vi "importExcel.vi"(1 "RANGE":string="A1:D2", 2 "Path":path) -> (0 "Excel Data":dbl[][](array[numeric]))   [LabVIEW 2019]
panel:
  in  "Array - Used for data type":string[][](array[string])
  in  "Excel._Worksheet 2":refnum<k7>
  in  "Excel._Application":refnum<k7>
  # "Filepath to Excel file"
  # "Specify range to import from Excel"
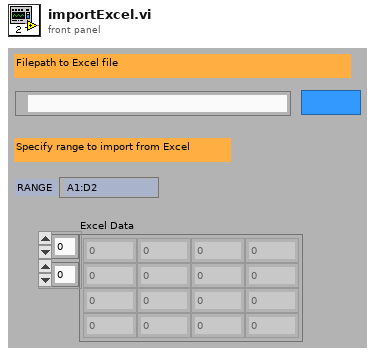
[diagram p1: front panel]
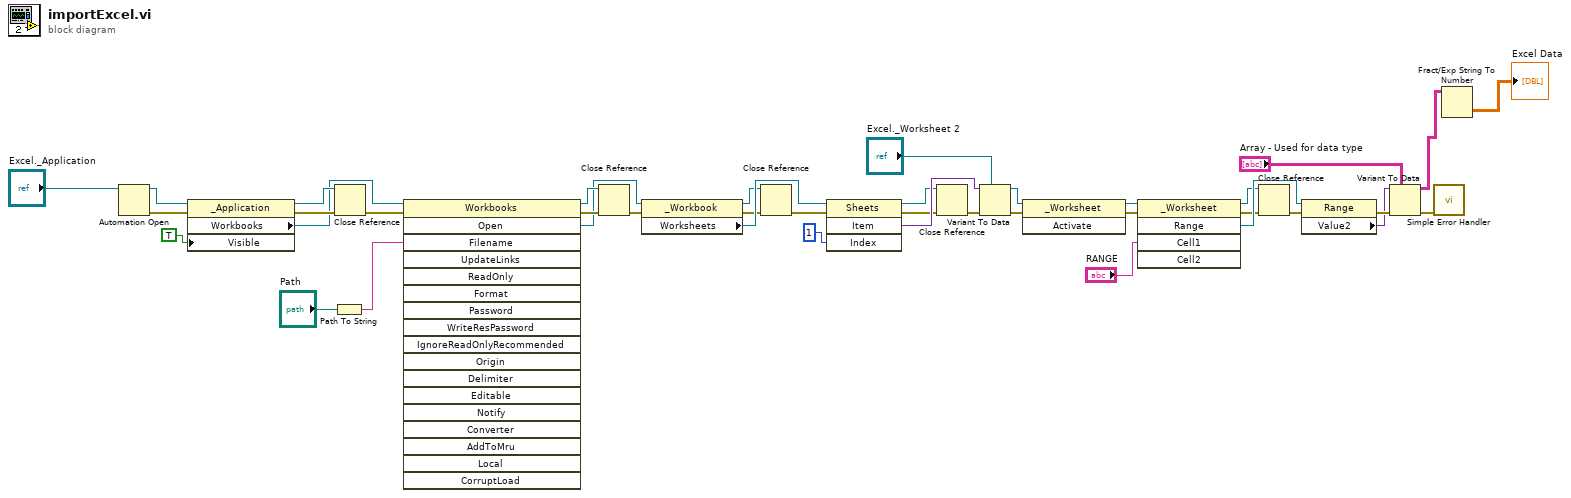
[diagram p0: block diagram]
diagram:
  n1 = Automation Open(Automation Refnum="Excel._Application") -> (Automation Refnum=w4:refnum<k7>, error out=w26:errorcluster)  [unwired: 3 in]
  n2 = property class="_Application"(reference=w4, error in=w26, "Visible"=TRUE) -> (reference out=w24:refnum<k7>, error out=w20:errorcluster, "Workbooks"=w11:refnum<k7>)
  n3 = Path To String(path="Path") -> (string=w38:string)
  n4 = Close Reference(reference=w24, error in (no error)=w20) -> (error out=w19:errorcluster)
  n5 = invoke class="Workbooks" method="Open"(reference=w11, error in=w19, "Filename"=w38) -> (reference out=w23:refnum<k7>, error out=w18:errorcluster, "Open"=w10:refnum<k7>)  [unwired: 15 in, 15 out]
  n6 = Close Reference(reference=w23, error in (no error)=w18) -> (error out=w17:errorcluster)
  n7 = property class="_Workbook"(reference=w10, error in=w17) -> (reference out=w22:refnum<k7>, error out=w16:errorcluster, "Worksheets"=w34:refnum<k7>)
  n8 = Close Reference(reference=w22, error in (no error)=w16) -> (error out=w15:errorcluster)
  n9 = invoke class="Sheets" method="Item"(reference=w34, error in=w15, "Index"=1) -> (reference out=w21:refnum<k7>, error out=w14:errorcluster, "Item"=w35:variant)  [unwired: 1 in, 1 out]
  n10 = Close Reference(reference=w21, error in (no error)=w14) -> (error out=w13:errorcluster)
  n11 = Variant To Data(error in=w13, type="Excel._Worksheet 2", Variant=w35) -> (data=w5:refnum<k7>, error out=w25:errorcluster)
  n12 = invoke class="_Worksheet" method="Activate"(reference=w5, error in=w25) -> (reference out=w3:refnum<k7>, error out=w12:errorcluster)  [unwired: 1 in, 1 out]
  n13 = invoke class="_Worksheet" method="Range"(reference=w3, error in=w12, "Cell1"="RANGE") -> (reference out=w9:refnum<k7>, error out=w8:errorcluster, "Range"=w29:refnum<k7>)  [unwired: 2 in, 2 out]
  n14 = Close Reference(reference=w9, error in (no error)=w8) -> (error out=w7:errorcluster)
  n15 = property class="Range"(reference=w29, error in=w7) -> (error out=w31:errorcluster, "Value2"=w30:variant)  [unwired: 1 out]
  n16 = Variant To Data(error in=w31, type="Array - Used for data type", Variant=w30) -> (data=w2:string[][], error out=w6:errorcluster)
  n17 = call <vilib>:"Simple Error Handler.vi"("error in (no error)"=w6) -> ()  [unwired: 4 in, 5 out]
  n18 = Fract/Exp String To Number(string=w2) -> (number=→"Excel Data":dbl[][])  [unwired: 3 in, 1 out]
